vi "Show_Save_Load_XY_Data.vi"(2 "1D Array X":dbl[](array[numeric]) format="%.6f", 3 "1D Array Y":dbl[](array[numeric]) format="%.6f", 5 "error in":errorcluster, 6 "No. of digits X":i32=3 min=0, 7 "No. of digits Y":i16=2 min=0, 9 "Autoscale":bool, 11 "Names":string[](array[string])) -> (19 "error out":errorcluster)   [LabVIEW 2026]
doc: "This VI displays XY data in an XY Graph. If 1D Array X is an empty array, N X values are calculated with N = Size of 1D Array Y and Delta X = 1. No. of digits determines the resolution of Table and XY Graph. Data can be saved or loaded and a screen copy can be saved as JPG.\n\nIf data (1D Array X, 1D Array Y) are sent to the VI via the corresponding connectors, the VI will display the corresponding graphics after being called. To load data at runtime, press the Load data button. A dialog will pop up where a data file to open can be selected. The VI can read data in GCSArray, GCSTable and simple ASCII column format. Autoscale can be switched on or off. If Autoscale is off, the Y axis of the graph is scaled from 0-10. \n\nPress Save data to save data (file header and numerical data). Data will be saved in GCS Array format. The file header will contain information given in X axis name, Y axis name and Remarks. With Save panel a screen copy of this VI can be saved as a JPG file. XY Graph will show the Y values over corresponding X values. Table contains the numerical values for X and Y. Press Exit to stop execution of this VI."
uses:
  <vilib>/Analysis/3filter.llb/Butterworth Filter (DBL).vi
  <vilib>/Analysis/NI_AALBase.lvlib
panel:
  in  "Filter options":T1={"Filter type"=enum."Lowpass", "Order"=5, "Sampling f"=1000.0, "High cutoff f"=0.45000000000000007, "Low cutoff f"=40.0} {"Low cutoff f" format="%0.4f"; "High cutoff f" format="%0.2f"; "Sampling f" format="%0.2f"}
  in  "Filter":bool
  out "File path":path=path "no path"
  out "error":bool
  in  "Save jpg":bool
  in  "Remarks":string
  in  "Y axis name":string
  in  "X axis name":string
  in  "Redraw":bool
  in  "Next frame":i32
  in  "Exit":bool
  in  "Save data":bool
  in  "Load data":bool
  out "Table":string[][](table)
  out "XY Graph":cluster{"1D Array X":dbl[], "1D Array Y":dbl[]}(graph)
  # "This vi displays XY data in a XY Graph. If \"1D Array X\" is an empty array, N X values are calculated with N = Size of \"1D Array Y\"\nand Delta X = 1. No. of digits determines resolution of Table and XY Graph. Data can be saved or loaded and screen copy can \nbe saved as JPG."
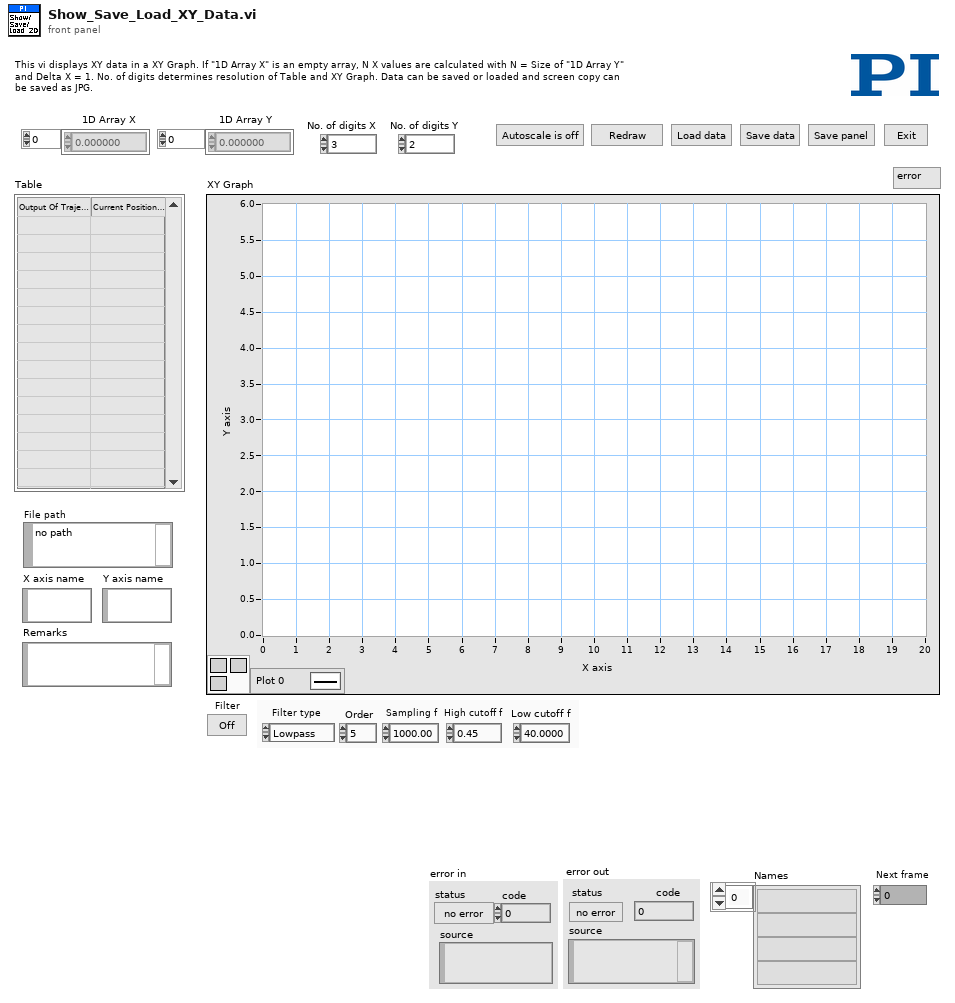
[diagram p1: front panel]
types:
  T1 = cluster{"Filter type":enum32{"Lowpass", "Highpass", "Bandpass", "Bandstop"}, "Order":i32, "Sampling f":dbl, "High cutoff f":dbl, "Low cutoff f":dbl}
  T2 = cluster{"XName":string, "YName":string, "ZName":string}
  T3 = cluster{"Separator":string, "Remarks":string, "NDim":i32}
  T4 = cluster{"Read (F)/ Write":bool, "Path":path, "Datastream":string, "ArrayName":string}
  T5 = cluster{"Filter type":bool, "Order":bool, "Sampling f":bool, "High cutoff f":bool, "Low cutoff f":bool}
  T6 = typedef "GCSArray_header.ctl" = cluster{"Identifier":string, "Version":i32, "Remark":string, "Dimension":i32, "Type":enum16{"Matrix", "Table"}, "Separator":u8, "NData":i32, "NData%":i32[], "Name%":string[], "Start%":dbl[], "End%":dbl[], "Delta%":dbl[], "SampleTime":dbl, "TransmittedUnit%":string[], "DisplayedUnit%":string[], "RatioNominator%":dbl[], "RatioDenominator%":dbl[]}
  T7 = enum32{"Lowpass", "Highpass", "Bandpass", "Bandstop"}
  T8 = typedef "imagedata.ctl" = cluster{"image type":i32, "image depth":i32, "image":u8[], "mask":u8[], "colors":u32[], "Rectangle":cluster{"left":i16, "top":i16, "right":i16, "bottom":i16}}
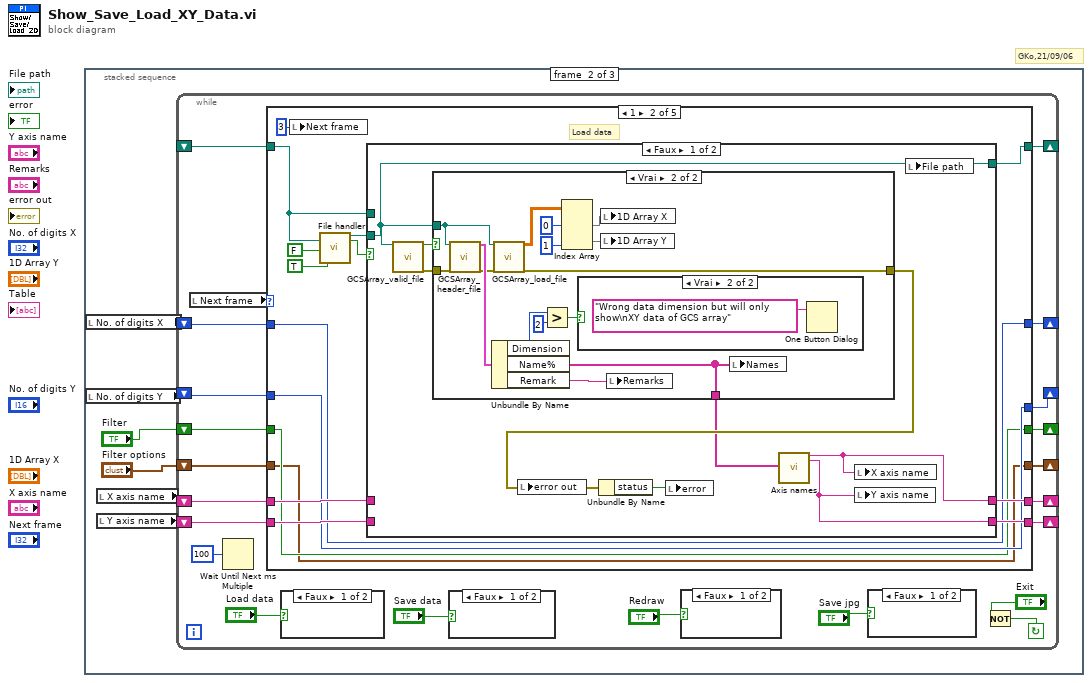
[diagram p0: block diagram]
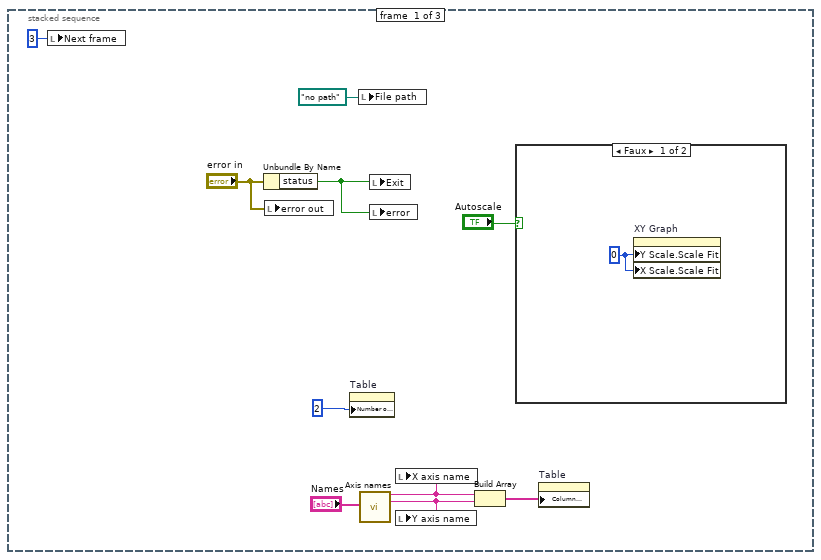
[diagram p2: hidden frame]
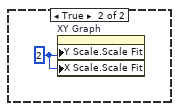
[diagram p3: hidden frame]
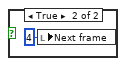
[diagram p4: hidden frame]
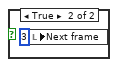
[diagram p5: hidden frame]
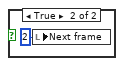
[diagram p6: hidden frame]
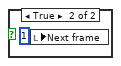
[diagram p7: hidden frame]
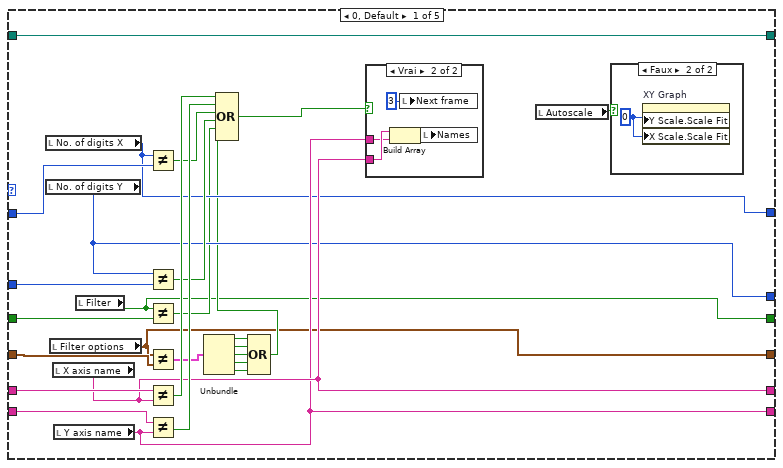
[diagram p8: hidden frame]
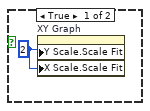
[diagram p10: hidden frame]
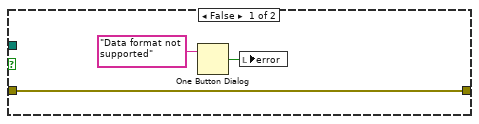
[diagram p11: hidden frame]
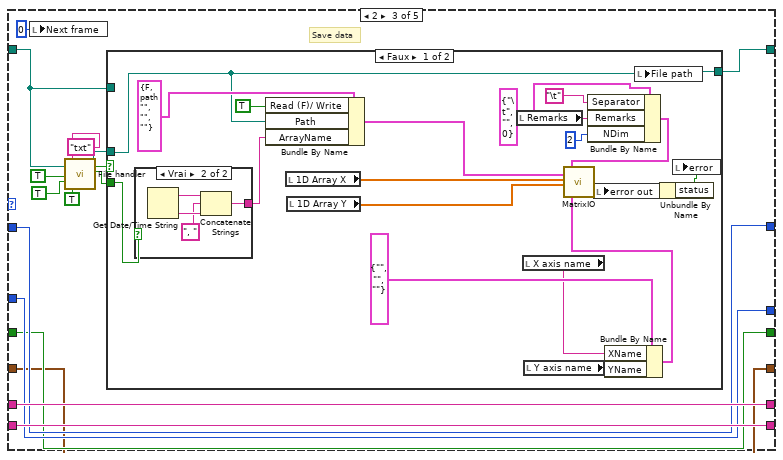
[diagram p14: hidden frame]
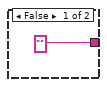
[diagram p15: hidden frame]
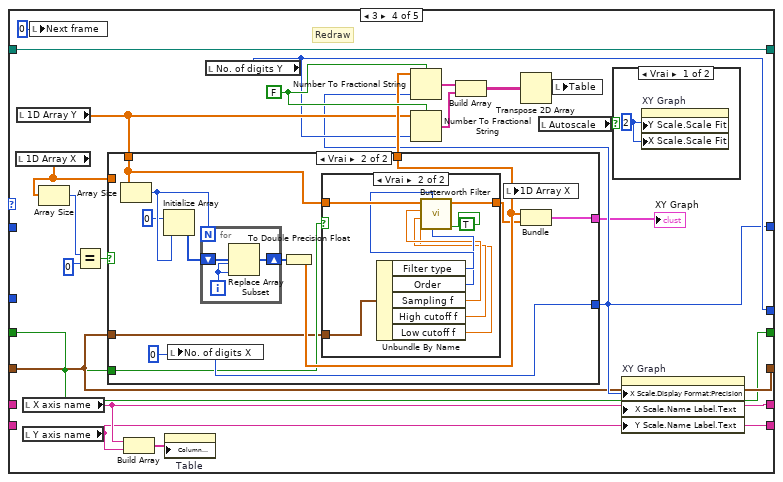
[diagram p17: hidden frame]
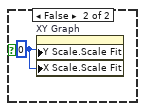
[diagram p18: hidden frame]
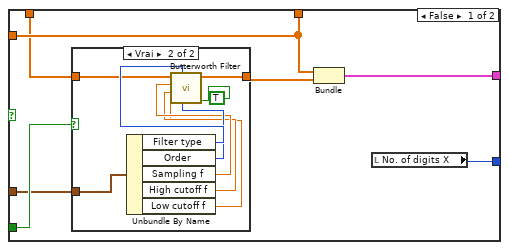
[diagram p19: hidden frame]
diagram:
  # "GKo,21/09/06"
  n1 = stacked-sequence {
    frame #0 {
      n2 = local write "Next frame"(3 ("Next frame")) -> ()
      n3 = Unbundle By Name("error in") -> ("status"=w3:bool)
      n4 = local write "error out"("error in") -> ()
      n5 = property on="Table" class="Tbl (strict)"("Number of Columns"=u32 2 ("Write Attribute")) -> ()  [unwired: 2 in, 2 out]
      n6 = local write "File path"(path "no path" ("File path")) -> ()
      n7 = call "Axis names.vi"("Names"="Names") -> ("X axis name"=w5:string, "Y axis name"=w4:string)  [unwired: 17 out]
      n8 = local write "Exit"(w3) -> ()
      n9 = local write "error"(w3) -> ()
      n10 = local write "X axis name"(w5) -> ()
      n11 = local write "Y axis name"(w4) -> ()
      n12 = Build Array(w5, w4) -> (w7:string[])
      n13 = case shown="Faux" "Autoscale" {
        frame False {
          w11 = u8 0 ("Write Attribute")
          n14 = property on="XY Graph" class="GraphXY (strict)"("Y Scale.Scale Fit"=w11, "X Scale.Scale Fit"=w11) -> ()  [unwired: 2 in, 2 out]
        }
        frame True {
          w12 = u8 2 ("Write Attribute")
          n15 = property on="XY Graph" class="GraphXY (strict)"("Y Scale.Scale Fit"=w12, "X Scale.Scale Fit"=w12) -> ()  [unwired: 2 in, 2 out]
        }
      }
      n16 = property on="Table" class="Tbl (strict)"("Column Header Strings[]"=w7) -> ()  [unwired: 2 in, 2 out]
    }
    frame #1 {
      n17 = local read "No. of digits X"() -> (w16:i32)
      n18 = local read "No. of digits Y"() -> (w15:i16)
      n19 = local read "X axis name"() -> (w18:string)
      n20 = local read "Y axis name"() -> (w17:string)
      n21 = while {
        shift-left: w15 -> [w26]
        shift-right: [w23] -> _
        shift-left: w16 -> [w25]
        shift-right: [w24] -> _
        shift-left: w17 -> [w29]
        shift-right: [w27] -> _
        shift-left: w18 -> [w30]
        shift-right: [w28] -> _
        shift-left: _ -> [w32]
        shift-right: [w33] -> _
        shift-right: [w19] -> _
        shift-left: "Filter" -> [w22]
        shift-right: [w20] -> _
        shift-left: "Filter options" -> [w21]
        stop <- w39 continue-if-true
        n22 = local read "Next frame"() -> (w38:i32)
        n23 = Wait Until Next ms Multiple(millisecond multiple=u32 100) -> ()  [unwired: 1 out]
        n24 = case shown="1" w38 {
          tunnel: [w70 w81 w126 w171 w238] -> w33
          tunnel: w32 -> [w70 w80 w125 w171 w231]
          tunnel: w30 -> [w67 w86 w132 _ w235]
          tunnel: w29 -> [w66 w85 w131 _ w234]
          tunnel: [w64 w88 w132 w170 w235] -> w28
          tunnel: [w63 w87 w131 w169 w234] -> w27
          tunnel: w26 -> [w58 w83 w129 _ w232]
          tunnel: w25 -> [w60 w84 w130 _ w233]
          tunnel: [w59 w84 w130 w167 w233] -> w24
          tunnel: [w57 w83 w129 w168 w232] -> w23
          tunnel: w22 -> [w55 w79 w124 w164 w230]
          tunnel: w21 -> [w54 w78 w123 w165 w229]
          tunnel: [w46 w78 w123 w165 w229] -> w20
          tunnel: [w45 w79 w124 w164 w230] -> w19
          frame 0, Default {
            n25 = local read "No. of digits X"() -> (w59:i32)
            n26 = local read "No. of digits Y"() -> (w57:i16)
            n27 = local read "Filter options"() -> (w46:T1)
            n28 = local read "X axis name"() -> (w64:string)
            n29 = local read "Y axis name"() -> (w63:string)
            n30 = local read "Filter"() -> (w45:bool)
            n31 = Not Equal?(x=w59, y=w60) -> (x != y?=w62:bool)
            n32 = Not Equal?(x=w57, y=w58) -> (x != y?=w61:bool)
            n33 = Not Equal?(x=w45, y=w55) -> (x != y?=w56:bool)
            n34 = Not Equal?(x=w46, y=w54) -> (x != y?=w53:T5)
            n35 = Not Equal?(x=w67, y=w64) -> (x != y?=w69:bool)
            n36 = Not Equal?(x=w66, y=w63) -> (x != y?=w68:bool)
            n37 = Unbundle(w53) -> ("Filter type"=w52:bool, "Order"=w51:bool, "Sampling f"=w50:bool, "High cutoff f"=w49:bool, "Low cutoff f"=w48:bool)
            n38 = Compound Arithmetic op=OR(w52, w51, w50, w49, w48) -> (w47:bool)
            n39 = Compound Arithmetic op=OR(w69, w68, w62, w61, w56, w47) -> (w65:bool)
            n40 = case shown="Vrai" w65 {
              tunnel: w64 -> [_ w75]
              tunnel: w63 -> [_ w74]
              frame False {
              }
              frame True {
                n41 = Build Array(w75, w74) -> (w73:string[])
                n42 = local write "Next frame"(3 ("Next frame")) -> ()
                n43 = local write "Names"(w73) -> ()
              }
            }
            n44 = local read "Autoscale"() -> (w71:bool)
            n45 = case shown="Faux" w71 {
              frame True {
                w76 = u8 2 ("Write Attribute")
                n46 = property on="XY Graph" class="GraphXY (strict)"("Y Scale.Scale Fit"=w76, "X Scale.Scale Fit"=w76) -> ()  [unwired: 2 in, 2 out]
              }
              frame False {
                w77 = u8 0 ("Write Attribute")
                n47 = property on="XY Graph" class="GraphXY (strict)"("Y Scale.Scale Fit"=w77, "X Scale.Scale Fit"=w77) -> ()  [unwired: 2 in, 2 out]
              }
            }
          }
          frame 1 {
            # "Load data"
            n48 = local write "Next frame"(3 ("Next frame")) -> ()
            n49 = call "File handler.vi"("Path in"=w80, "Read (F) or write (T)?"=FALSE, "With dialog?"=TRUE ("With dialog")) -> ("Path out"=w82:path, "Cancelled?"=w90:bool)  [unwired: 3 in, 12 out]
            n50 = case shown="Faux" w90 {
              tunnel: w82 -> [w93 _]
              tunnel: [w100 w122] -> w88
              tunnel: [w99 w121] -> w87
              tunnel: w86 -> [_ w122]
              tunnel: w85 -> [_ w121]
              tunnel: [w93 w120] -> w81
              tunnel: w80 -> [_ w120]
              frame False {
                n51 = call "GCSArray_valid_file.vi"("GCS Array Filepath"=w93) -> ("Is valid?"=w95:bool, "error out"=w98:errorcluster)  [unwired: 17 in]
                n52 = case shown="Vrai" w95 {
                  tunnel: w98 -> [w103 w118]
                  tunnel: [w103 w117] -> w96
                  tunnel: w93 -> [_ w107]
                  tunnel: [_ w108] -> w94
                  frame False {
                    n53 = One Button Dialog(message="Data format not supported") -> (true=w101:bool)  [unwired: 1 out]
                    n54 = local write "error"(w101) -> ()
                  }
                  frame True {
                    n55 = call "GCSArray_header_file.vi"("GCS Array Filepath"=w107, "error in (no error)"=w118) -> ("GCSArray Header"=w110:T6, "error out"=w104:errorcluster)  [unwired: 16 in]
                    n56 = Unbundle By Name(w110) -> ("Dimension"=w111:i32, "Name%"=w108:string[], "Remark"=w106:string)
                    n57 = call "GCSArray_load_file.vi"("GCS Array Filepath"=w107, "error in (no error)"=w104) -> ("GCSArray data"=w114:dbl[][], "error out"=w117:errorcluster)  [unwired: 16 in]
                    n58 = Greater?(x=w111, y=2) -> (0:w105:bool)
                    n59 = Index Array(array=w114, index (col) #1=0 ("disabled index (col)"), index (col) #2=1 ("index (col)")) -> (element #1=w116:dbl[], element #2=w115:dbl[])  [unwired: 2 in]
                    n60 = case shown="Vrai" w105 {
                      frame False {
                      }
                      frame True {
                        n61 = One Button Dialog(message="Wrong data dimension but will only show\nXY data of GCS array") -> ()  [unwired: 2 out]
                      }
                    }
                    n62 = local write "1D Array X"(w116) -> ()
                    n63 = local write "1D Array Y"(w115) -> ()
                    n64 = local write "Remarks"(w106) -> ()
                    n65 = local write "Names"(w108) -> ()
                  }
                }
                n66 = local write "error out"(w96) -> ()
                n67 = Unbundle By Name(w96) -> ("status"=w97:bool)
                n68 = local write "error"(w97) -> ()
                n69 = call "Axis names.vi"("Names"=w94) -> ("X axis name"=w100:string, "Y axis name"=w99:string)  [unwired: 17 out]
                n70 = local write "X axis name"(w100) -> ()
                n71 = local write "Y axis name"(w99) -> ()
                n72 = local write "File path"(w93) -> ()
              }
              frame True {
              }
            }
          }
          frame 2 {
            # "Save data"
            n73 = local write "Next frame"(0 ("Next frame")) -> ()
            n74 = call "File handler.vi"("Path in"=w125, "Read (F) or write (T)?"=TRUE ("New File?"), "Write new File?"=TRUE, "Extension"="txt", "With dialog?"=TRUE ("With dialog")) -> ("Path out"=w127:path, "Cancelled?"=w137:bool, "Data added?"=w134:bool)  [unwired: 1 in, 11 out]
            n75 = case shown="Faux" w137 {
              tunnel: w127 -> [w140 _]
              tunnel: w134 -> [w144 _]
              tunnel: [w140 w163] -> w126
              tunnel: w125 -> [_ w163]
              frame False {
                n76 = case shown="Vrai" w144 {
                  tunnel: ["" ("ArrayName") w159] -> w143
                  frame False {
                  }
                  frame True {
                    n77 = Get Date/Time String() -> (date string=w162:string, time string=w161:string)  [unwired: 3 out]
                    n78 = Concatenate Strings(w162, ", " ("Substring"), w161) -> (w159:string)
                  }
                }
                n79 = Bundle By Name(cluster=T4 {"Read (F)/ Write"=FALSE, "Path"=path "", "Datastream"="", "ArrayName"=""} ("IOSource"), "Read (F)/ Write"=TRUE, "Path"=w140, "ArrayName"=w143) -> (w153:T4)
                n80 = local read "1D Array X"() -> (w156:dbl[])
                n81 = local read "1D Array Y"() -> (w157:dbl[])
                n82 = local read "Remarks"() -> (w151:string)
                n83 = local read "X axis name"() -> (w147:string)
                n84 = local read "Y axis name"() -> (w146:string)
                n85 = Bundle By Name(cluster=T3 {"Separator"="\t", "Remarks"="", "NDim"=0} ("Header in"), "Separator"="\t", "Remarks"=w151, "NDim"=2) -> (w149:T3)
                n86 = Bundle By Name(cluster=T2 {"XName"="", "YName"="", "ZName"=""} ("Data names"), "XName"=w147, "YName"=w146) -> (w145:T2)
                n87 = call "MatrixIO.vi"("IOSource"=w153, "XArray in"=w156, "YArray in"=w157, "Header in"=w149, "Data names"=w145) -> ("error out"=w142:errorcluster)  [unwired: 2 in, 12 out]
                n88 = local write "error out"(w142) -> ()
                n89 = local write "File path"(w140) -> ()
                n90 = Unbundle By Name(w142) -> ("status"=w141:bool)
                n91 = local write "error"(w141) -> ()
              }
              frame True {
              }
            }
          }
          frame 3 {
            w182 = FALSE ("use system decimal point (T)")
            # "Redraw"
            n92 = local read "1D Array X"() -> (w174:dbl[])
            n93 = local read "1D Array Y"() -> (w179:dbl[])
            n94 = local read "X axis name"() -> (w170:string)
            n95 = local read "Y axis name"() -> (w169:string)
            n96 = local write "Next frame"(0 ("Next frame")) -> ()
            n97 = Array Size(array=w174) -> (size(s)=w177:i32)
            n98 = Equal?(x=w177, y=0) -> (x = y?=w175:bool)
            n99 = case shown="Vrai" w175 {
              tunnel: [w194 w212] -> w166
              tunnel: [w193 w211] -> w167
              tunnel: [w192 w209] -> w181
              tunnel: w179 -> [w189 w208]
              tunnel: w174 -> [w192 _]
              tunnel: w164 -> [w190 w206]
              tunnel: w165 -> [w188 w205]
              frame False {
                n100 = case shown="Vrai" w190 {
                  tunnel: w189 -> [w195 w196]
                  tunnel: [w195 w203] -> w191
                  tunnel: w188 -> [_ w197]
                  frame False {
                  }
                  frame True {
                    n101 = Unbundle By Name(w197) -> ("Filter type"=w202:T7, "Order"=w201:i32, "Sampling f"=w200:dbl, "High cutoff f"=w199:dbl, "Low cutoff f"=w198:dbl)
                    n102 = call-poly <vilib>:"Butterworth Filter.vi"("init/cont (init:F)"=TRUE, "order"=w201, "filter type"=w202, "low cutoff freq: fl"=w198, "high cutoff freq: fh"=w199, "sampling freq: fs"=w200, "X"=w196) -> ("Filtered X"=w203:dbl[])  [unwired: 2 out]
                  }
                }
                n103 = Bundle("1D Array X"=w192, "Filtered X"=w191) -> (w194:cluster{"1D Array X":dbl[], "Filtered X":dbl[]})  [unwired: 1 out]
                n104 = local read "No. of digits X"() -> (w193:i32)
              }
              frame True {
                w211 = 0
                n105 = Array Size(array=w208) -> (size(s)=w214:i32)
                n106 = Initialize Array(0 ("Element Data"), w214) -> (w215:i32[])
                n107 = local write "No. of digits X"(w211) -> ()
                n108 = for {
                  N: w214 -> [_]
                  shift-right: [w226] -> w210
                  shift-left: w215 -> [w228]
                  i -> [w227]
                  n109 = Replace Array Subset(array=w228, new element=w227, index=w227) -> (w226:i32[])
                }
                n110 = To Double Precision Float(number=w210) -> (double precision float=w209:dbl[])
                n111 = case shown="Vrai" w206 {
                  tunnel: w208 -> [w216 w225]
                  tunnel: [w216 w223] -> w207
                  tunnel: w205 -> [_ w217]
                  frame False {
                  }
                  frame True {
                    n112 = Unbundle By Name(w217) -> ("Filter type"=w222:T7, "Order"=w221:i32, "Sampling f"=w220:dbl, "High cutoff f"=w219:dbl, "Low cutoff f"=w218:dbl)
                    n113 = call-poly <vilib>:"Butterworth Filter.vi"("init/cont (init:F)"=TRUE, "order"=w221, "filter type"=w222, "low cutoff freq: fl"=w218, "high cutoff freq: fh"=w219, "sampling freq: fs"=w220, "X"=w225) -> ("Filtered X"=w223:dbl[])  [unwired: 2 out]
                  }
                }
                n114 = local write "1D Array X"(w209) -> ()
                n115 = Bundle(w209, "Filtered X"=w207) -> (w212:cluster{dbl[], "Filtered X":dbl[]})  [unwired: 1 out]
              }
            }
            "XY Graph" <- w166
            n116 = Build Array(w170, w169) -> (w172:string[])
            n117 = property on="Table" class="Tbl (strict)"("Column Header Strings[]"=w172) -> ()  [unwired: 2 in, 2 out]
            n118 = local read "No. of digits Y"() -> (w168:i16)
            n119 = Number To Fractional String(use system decimal point (T)=w182, number=w181, precision (6)=w167) -> (F-format string=w185:string[])  [unwired: 1 out]
            n120 = Number To Fractional String(use system decimal point (T)=w182, number=w179, precision (6)=w168) -> (F-format string=w184:string[])  [unwired: 1 out]
            n121 = Build Array(w185, w184) -> (w183:string[][])
            n122 = Transpose 2D Array(2D array=w183) -> (transposed array=w178:string[][])
            n123 = local read "Autoscale"() -> (w173:bool)
            n124 = local write "Table"(w178) -> ()
            n125 = case shown="Vrai" w173 {
              frame True {
                w186 = u8 2 ("Write Attribute")
                n126 = property on="XY Graph" class="GraphXY (strict)"("Y Scale.Scale Fit"=w186, "X Scale.Scale Fit"=w186) -> ()  [unwired: 2 in, 2 out]
              }
              frame False {
                w187 = u8 0 ("Write Attribute")
                n127 = property on="XY Graph" class="GraphXY (strict)"("Y Scale.Scale Fit"=w187, "X Scale.Scale Fit"=w187) -> ()  [unwired: 2 in, 2 out]
              }
            }
            n128 = property on="XY Graph" class="GraphXY (strict)"("X Scale.Display Format:Precision"=w167, "X Scale.Name Label.Text"=w170, "Y Scale.Name Label.Text"=w169) -> ()  [unwired: 2 in, 2 out]
          }
          frame 4 {
            # "Save jpg"
            n129 = local write "Next frame"(0 ("Next frame")) -> ()
            n130 = call "File handler.vi"("Path in"=w231, "Read (F) or write (T)?"=TRUE ("New File?"), "Write new File?"=TRUE, "Extension"="jpg", "With dialog?"=TRUE ("With dialog")) -> ("Path out"=w237:path, "Cancelled?"=w243:bool, "Data added?"=w240:bool)  [unwired: 1 in, 11 out]
            n131 = case shown="Faux" w243 {
              tunnel: w237 -> [w248 _]
              tunnel: w240 -> [_ _]
              tunnel: [w250 w254] -> w238
              tunnel: w231 -> [_ w254]
              frame False {
                n132 = control-ref of="This VI"() -> (w246:refnum<vi>)
                n133 = invoke class="VI" method="FA.ObtImage"(reference=w246, "visible area only"=TRUE, "image depth"=24) -> (error out=w249:errorcluster, "image data"=w247:T8)  [unwired: 3 in, 4 out]
                n134 = call <vilib>:"Write JPEG File.vi"("error in (no error)"=w249, "image data"=w247, "path to JPEG file"=w248) -> ("error out"=w245:errorcluster, "path"=w250:path)  [unwired: 7 in]
                n135 = local write "error out"(w245) -> ()
                n136 = Unbundle By Name(w245) -> ("status"=w251:bool)
                n137 = local write "error"(w251) -> ()
                n138 = local write "File path"(w250) -> ()
              }
              frame True {
              }
            }
          }
        }
        n139 = case shown="Faux" "Load data" {
          frame False {
          }
          frame True {
            n140 = local write "Next frame"(1) -> ()
          }
        }
        n141 = case shown="Faux" "Save data" {
          frame False {
          }
          frame True {
            n142 = local write "Next frame"(2) -> ()
          }
        }
        n143 = case shown="Faux" "Redraw" {
          frame False {
          }
          frame True {
            n144 = local write "Next frame"(3 ("Next frame")) -> ()
          }
        }
        n145 = case shown="Faux" "Save jpg" {
          frame False {
          }
          frame True {
            n146 = local write "Next frame"(4 ("Next frame")) -> ()
          }
        }
        n147 = Not(x="Exit") -> (.not. x?=w39:bool)
      }
    }
    frame #2 {
      n148 = local write "Exit"(FALSE ("stop")) -> ()
    }
  }
